vi "check magnet series bounds.vi"(10 "Output Voltage Limit":dbl=5.0 min=0.0 max=10.0, 11 "Magnet Voltage Sequence":dbl[](array[numeric])) -> (3 "Magnet Voltage Sequence":dbl[](array[numeric]))   [LabVIEW 2014]
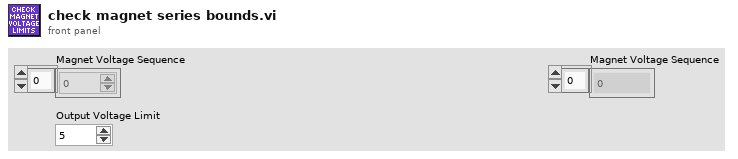
[diagram p1: front panel]
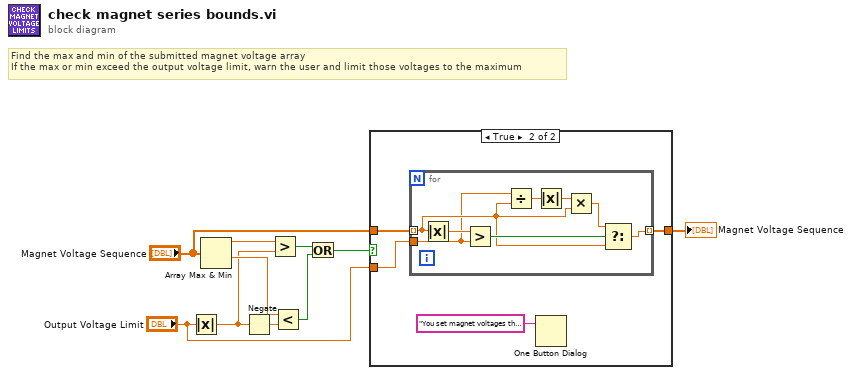
[diagram p0: block diagram]
diagram:
  # "Find the max and min of the submitted magnet voltage array\nIf the max or min exceed the output voltage limit, warn the user and limit those voltages to the maximum"
  n1 = Absolute Value(x="Output Voltage Limit") -> (abs(x)=w7:dbl)
  n2 = Array Max & Min(array="Magnet Voltage Sequence") -> (max value=w10:dbl, min value=w8:dbl)  [unwired: 2 out]
  n3 = Negate(x=w7) -> (-x=w9:dbl)
  n4 = Greater?(x=w10, y=w7) -> (0:w6:bool)
  n5 = Less?(x=w8, y=w9) -> (x < y?=w5:bool)
  n6 = Or(x=w6, y=w5) -> (x .or. y?=w4:bool)
  n7 = case shown="True" w4 {
    tunnel: "Magnet Voltage Sequence" -> [w11 w15]
    tunnel: [w11 w13] -> w2
    tunnel: "Output Voltage Limit" -> [_ w14]
    frame False {
    }
    frame True {
      n8 = for {
        tunnel: w15 -> [w17] mode=indexing
        tunnel: w14 -> [w16]
        tunnel: [w21] -> w13 mode=indexing
        n9 = Absolute Value(x=w17) -> (abs(x)=w23:dbl)
        n10 = Greater?(x=w23, y=w16) -> (0:w22:bool)
        n11 = Divide(x=w16, y=w17) -> (x/y=w18:dbl)
        n12 = Absolute Value(x=w18) -> (abs(x)=w20:dbl)
        n13 = Multiply(x=w20, y=w17) -> (x*y=w19:dbl)
        n14 = Select(t=w19, s=w22, f=w17) -> (s? t:f=w21:dbl)
      }
      n15 = One Button Dialog(message="You set magnet voltages that exceed the specified output voltage limit. The magnet voltages have been capped to your specified output limit.") -> ()  [unwired: 1 in, 1 out]
    }
  }
  "Magnet Voltage Sequence" <- w2
